vi "Create Class.vi"(8 "error in (no error)":errorcluster, 11 "Mock Class Generator in":refnum<class "Pure Mock Class Generator.lvclass">) -> (0 "error out":errorcluster, 3 "Mock Class Generator out":refnum<class "Pure Mock Class Generator.lvclass">)   [LabVIEW 2020, in "Pure Mock Class Generator.lvclass"]
uses:
  Pure Mock Class Generator.lvclass
  Pure Mock Class Generator.lvclass/Pure Mock Class Generator.ctl
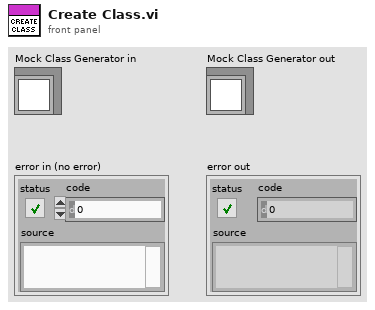
[diagram p1: front panel]
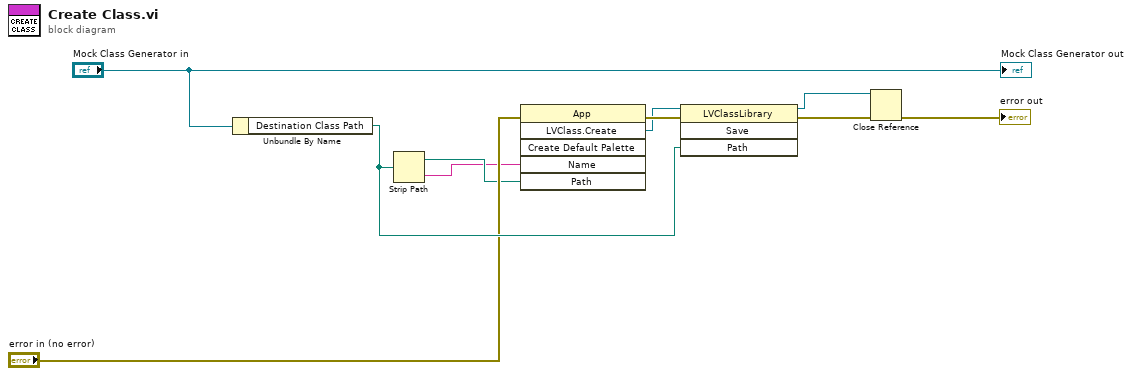
[diagram p0: block diagram]
diagram:
  n1 = Unbundle By Name("Mock Class Generator in") -> ("Destination Class Path"=w7:path)
  n2 = Strip Path(path=w7) -> (stripped path=w4:path, name=w3:string)
  n3 = invoke class="App" method="LVClass.Create"(error in="error in (no error)", "Name"=w3, "Path"=w4) -> (error out=w2:errorcluster, "LVClass.Create"=w1:refnum<vi>)  [unwired: 3 in, 4 out]
  n4 = invoke class="LVClassLibrary" method="Save"(reference=w1, error in=w2, "Path"=w7) -> (reference out=w9:refnum<vi>, error out=w6:errorcluster)  [unwired: 1 in, 2 out]
  n5 = Close Reference(reference=w9, error in (no error)=w6) -> (error out=→"error out":errorcluster)
  "Mock Class Generator out" <- "Mock Class Generator in"
